vi "ABB configure Bearing run.vi"() -> ()   [LabVIEW 2017]
uses:
  Temp error msg.ctl
  ABB global.vi
panel:
  in  "Temp error":T1="Error: Temperature measurement "
  in  "Category":T2(ring)
  in  "delete reading":bool
  in  "Add reading":bool
  in  "Temperature Measurement channels":i32(listbox)
  in  "Temperature Readings":i32(listbox)
  in  "Auto Reading":T3={"Thermal Stability (°C/hr)"=2.0, "Reading interval (mins)"=2.0}
  in  "Exit":bool
  # "Configure Bearing Run"
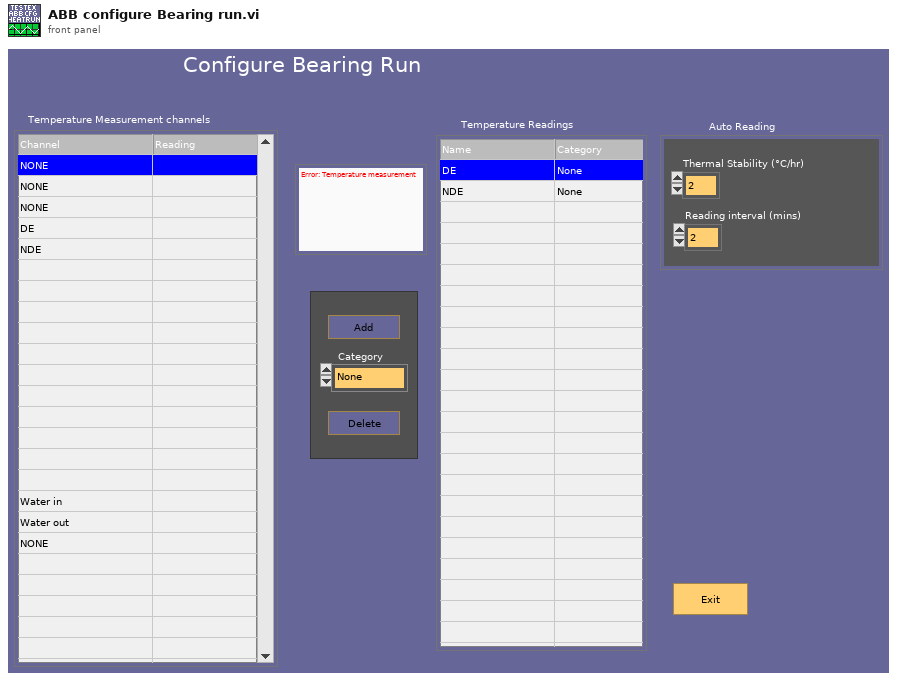
[diagram p1: front panel]
types:
  T1 = typedef "Temp error msg.ctl" = string
  T2 = enum16{"None", "Cool in", "Ambient", "DE", "NDE"}
  T3 = cluster{"Thermal Stability (°C/hr)":dbl, "Reading interval (mins)":dbl}
  T4 = cluster{"temp. alloc":i32[], "category":i32[], "Category names":string[], "Category none names":string[]}
  T5 = cluster{"Thermal Stability (%)":dbl, "Reading interval (mins)":dbl}
  T6 = cluster{"Simulate Norma":bool, "Norma 5000 Address":u8, "WebDaq IP Address":string, "Simulate cDAQ":bool}
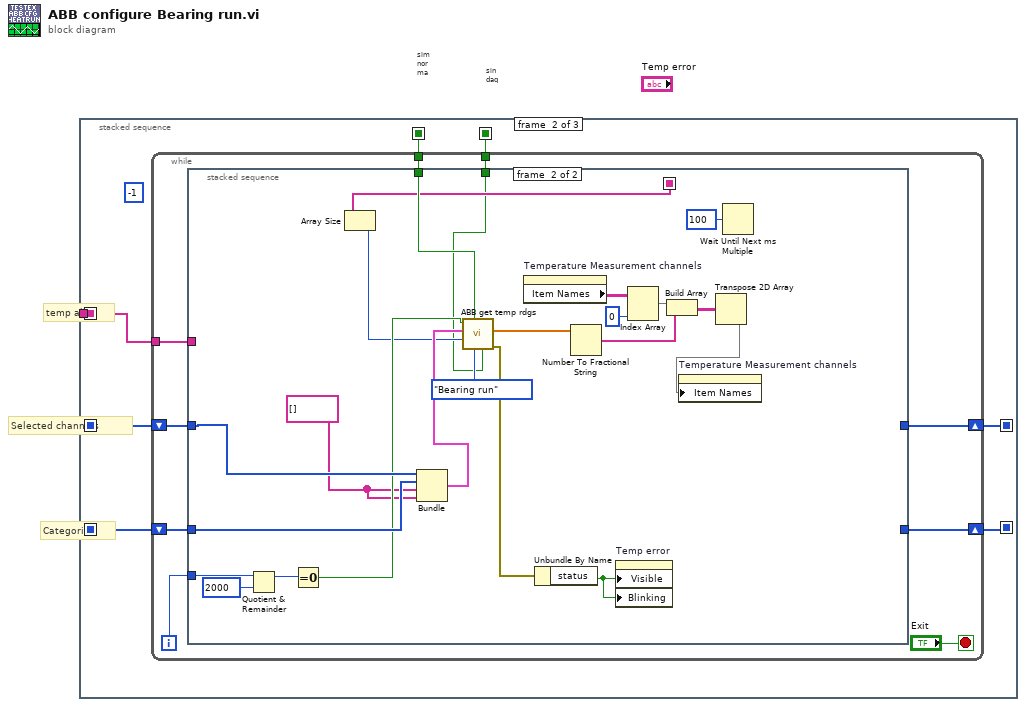
[diagram p0: block diagram]
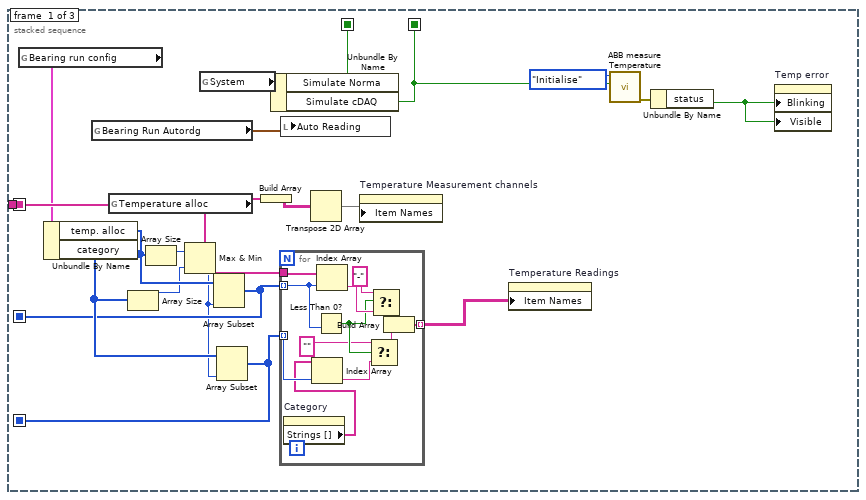
[diagram p2: hidden frame]
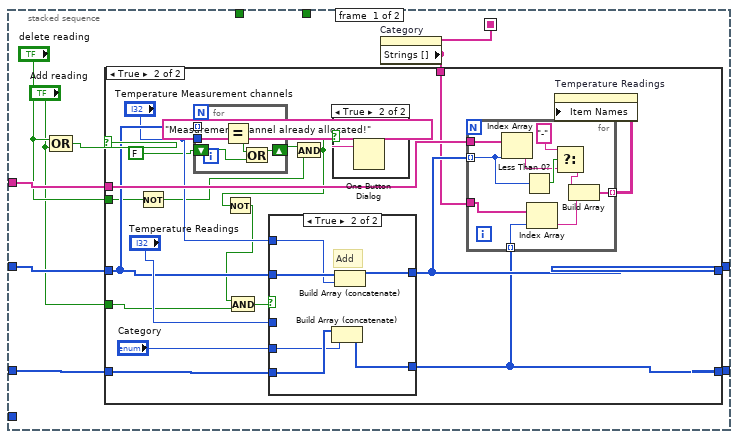
[diagram p3: hidden frame]
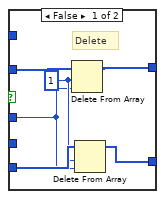
[diagram p6: hidden frame]
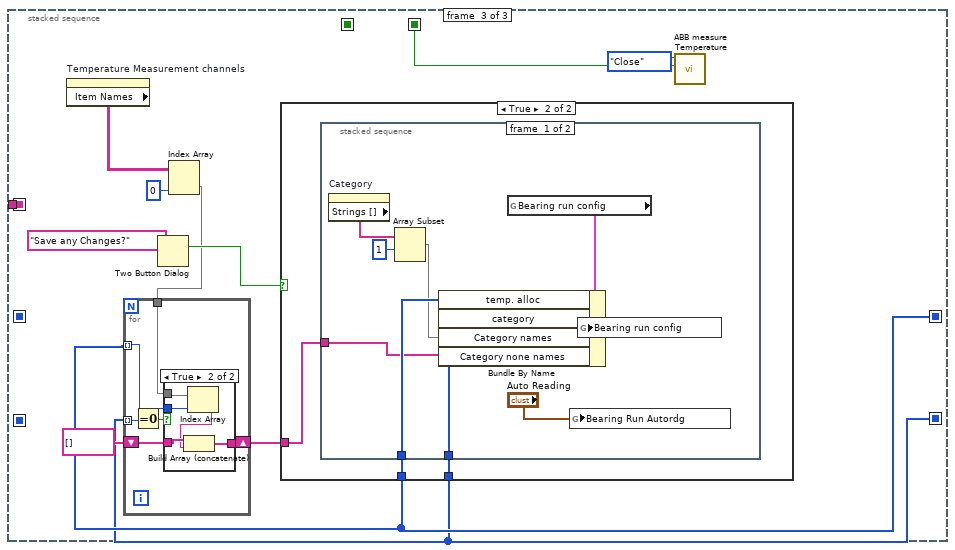
[diagram p7: hidden frame]
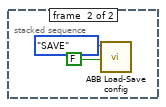
[diagram p10: hidden frame]
diagram:
  # "sin daq"
  # "sim norma"
  # "Categories"
  # "Selected channels"
  # "temp alloc"
  n1 = stacked-sequence {
    seq-local: [w7 _ _] -> [_ w38 _]
    seq-local: [_ w37 _] -> [_ _ w131]
    seq-local: [w16 _ _] -> [_ w36 _]
    seq-local: [w6 _ _] -> [_ w35 _]
    seq-local: [_ w34 _] -> [_ _ w130]
    seq-local: [w12 _ _] -> [_ w33 _]
    seq-local: [w4 _ _] -> [_ w32 w128]
    tunnel: [w16 _ _] -> _
    frame #0 {
      n2 = global read "ABB global.vi" "Bearing run config"() -> (w15:T4)
      n3 = Unbundle By Name(w15) -> ("temp. alloc"=w11:i32[], "category"=w10:i32[])
      n4 = global read "ABB global.vi" "Bearing Run Autordg"() -> (w19:T5)
      n5 = global read "ABB global.vi" "Temperature alloc"() -> (w16:string[])
      n6 = Array Size(array=w10) -> (size(s)=w8:i32)
      n7 = Array Size(array=w11) -> (size(s)=w9:i32)
      n8 = Max & Min(x=w9, y=w8) -> (min(x,y)=w5:i32)  [unwired: 1 out]
      n9 = global read "ABB global.vi" "System"() -> (w13:T6)
      n10 = Array Subset(array=w11, length=w5) -> (w7:i32[])  [unwired: 1 in]
      n11 = Array Subset(array=w10, length=w5) -> (w6:i32[])  [unwired: 1 in]
      n12 = Build Array(w16) -> (w18:string[][])
      n13 = Unbundle By Name(w13) -> ("Simulate Norma"=w12:bool, "Simulate cDAQ"=w4:bool)
      n14 = for {
        tunnel: w16 -> [w31]
        tunnel: w7 -> [w28] mode=indexing
        tunnel: w6 -> [w26] mode=indexing
        tunnel: [w21] -> w14 mode=indexing
        n15 = property on="Category" class="Enum (strict)"() -> ("Strings []"=w25:string[])  [unwired: 2 in, 2 out]
        n16 = Index Array(array=w25, index=w26) -> (element=w24:string)
        n17 = Less Than 0?(x=w28) -> (x < 0?=w27:bool)
        n18 = Index Array(array=w31, index=w28) -> (element=w29:string)
        n19 = Select(t="", s=w27, f=w24) -> (s? t:f=w23:string)
        n20 = Select(t="-", s=w27, f=w29) -> (s? t:f=w22:string)
        n21 = Build Array(w22, w23) -> (w21:string[])
      }
      n22 = local write "Auto Reading"(w19) -> ()
      n23 = Transpose 2D Array(2D array=w18) -> (transposed array=w17:string[][])
      n24 = property on="Temperature Measurement channels" class="MCListbox (strict)"("Item Names"=w17) -> ()  [unwired: 2 in, 2 out]
      n25 = property on="Temperature Readings" class="MCListbox (strict)"("Item Names"=w14) -> ()  [unwired: 2 in, 2 out]
      n26 = call "ABB measure Temperature.vi"("Simulate"=w4, "Mode"=enum16{"Initialise", "Read", "Close"}."Initialise") -> ("error out"=w2:errorcluster)  [unwired: 7 in, 2 out]
      n27 = Unbundle By Name(w2) -> ("status"=w1:bool)
      n28 = property on="Temp error" class="Str (strict)"("Blinking"=w1, "Visible"=w1) -> ()  [unwired: 2 in, 2 out]
    }
    frame #1 {
      (unwired) -1 ("Number Values")
      n29 = while {
        shift-right: [w45] -> w37
        shift-left: w38 -> [w46]
        tunnel: w36 -> [w44]
        shift-right: [w42] -> w34
        shift-left: w35 -> [w43]
        tunnel: w33 -> [w41]
        tunnel: w32 -> [w39]
        i -> [w40]
        stop <- "Exit" stop-if-true
        n30 = stacked-sequence {
          seq-local: [w48 _] -> [_ w110]
          tunnel: w46 -> [w56 w125]
          tunnel: [w55 _] -> w45
          tunnel: w44 -> [w54 _]
          tunnel: w43 -> [w51 w126]
          tunnel: [w50 _] -> w42
          tunnel: w41 -> [_ w127]
          tunnel: w40 -> [_ w115]
          tunnel: w39 -> [_ w107]
          frame #0 {
            n31 = Compound Arithmetic op=OR("delete reading", "Add reading") -> (w53:bool)
            n32 = property on="Category" class="Enum (strict)"() -> ("Strings []"=w48:string[])  [unwired: 2 in, 2 out]
            n33 = case shown="True" w53 {
              tunnel: w56 -> [w58 w69]
              tunnel: [w58 w73] -> w55
              tunnel: w54 -> [_ w76]
              tunnel: "delete reading" -> [_ w62]
              tunnel: w51 -> [w57 w72]
              tunnel: [w57 w71] -> w50
              tunnel: "Add reading" -> [_ w59]
              tunnel: w48 -> [_ w60]
              frame False {
              }
              frame True {
                n34 = Not(x=w62) -> (.not. x?=w61:bool)
                n35 = for {
                  tunnel: w69 -> [w82] mode=indexing
                  tunnel: "Temperature Measurement channels" -> [w81]
                  shift-right: [w78] -> w65
                  shift-left: FALSE -> [w79]
                  n36 = Equal?(x=w82, y=w81) -> (x = y?=w80:bool)
                  n37 = Or(x=w80, y=w79) -> (x .or. y?=w78:bool)
                }
                n38 = And(x=w65, y=w61) -> (x .and. y?=w63:bool)
                n39 = Not(x=w63) -> (.not. x?=w64:bool)
                n40 = And(x=w64, y=w59) -> (x .and. y?=w66:bool)
                n41 = case shown="True" w66 {
                  tunnel: "Category" -> [_ w90]
                  tunnel: "Temperature Measurement channels" -> [_ w92]
                  tunnel: w69 -> [w88 w94]
                  tunnel: [w87 w93] -> w73
                  tunnel: w72 -> [w86 w91]
                  tunnel: [w85 w89] -> w71
                  tunnel: "Temperature Readings" -> [w83 _]
                  frame False {
                    w84 = 1 ("length")
                    # "Delete"
                    n42 = Delete From Array(array=w88, length=w84, index=w83) -> (array with subset deleted=w87:i32[])  [unwired: 1 out]
                    n43 = Delete From Array(array=w86, length=w84, index=w83) -> (array with subset deleted=w85:i32[])  [unwired: 1 out]
                  }
                  frame True {
                    # "Add"
                    n44 = Build Array (concatenate)(w91, w90) -> (w89:i32[])
                    n45 = Build Array (concatenate)(w94, w92) -> (w93:i32[])
                  }
                }
                n46 = case shown="True" w63 {
                  frame False {
                  }
                  frame True {
                    n47 = One Button Dialog(message="Measurement channel already allocated!") -> ()  [unwired: 1 in, 1 out]
                  }
                }
                n48 = for {
                  tunnel: w73 -> [w103] mode=indexing
                  tunnel: w76 -> [w104]
                  tunnel: w60 -> [w98]
                  tunnel: w71 -> [w99] mode=indexing
                  tunnel: [w95] -> w75 mode=indexing
                  n49 = Index Array(array=w104, index=w103) -> (element=w101:string)
                  n50 = Less Than 0?(x=w103) -> (x < 0?=w102:bool)
                  n51 = Index Array(array=w98, index=w99) -> (element=w96:string)
                  n52 = Select(t="-", s=w102, f=w101) -> (s? t:f=w97:string)
                  n53 = Build Array(w97, w96) -> (w95:string[])
                }
                n54 = property on="Temperature Readings" class="MCListbox (strict)"("Item Names"=w75) -> ()  [unwired: 2 in, 2 out]
              }
            }
          }
          frame #1 {
            w111 = string[] []
            n55 = Quotient & Remainder(x=w115, y=2000) -> (x-y*floor(x/y)=w113:i32)  [unwired: 1 out]
            n56 = Equal To 0?(x=w113) -> (x = 0?=w112:bool)
            n57 = Array Size(array=w110) -> (size(s)=w109:i32)
            n58 = Bundle(w125, w126, w111, w111) -> (w124:cluster{i32[], i32[], string[], string[]})  [unwired: 1 in]
            n59 = call "ABB get temp rdgs.vi"("Sim daq"=w107, "sim type"=enum16{"Heat run", "Bearing run"}."Bearing run", "Simulate norma"=w127, "# categories"=w109, "run config"=w124, "start"=w112) -> ("error out"=w106:errorcluster, "Measured temps"=w123:dbl[])  [unwired: 2 in, 2 out]
            n60 = property on="Temperature Measurement channels" class="MCListbox (strict)"() -> ("Item Names"=w122:string[][])  [unwired: 2 in, 2 out]
            n61 = Unbundle By Name(w106) -> ("status"=w105:bool)
            n62 = Number To Fractional String(number=w123) -> (F-format string=w119:string[])  [unwired: 3 in]
            n63 = property on="Temp error" class="Str (strict)"("Visible"=w105, "Blinking"=w105) -> ()  [unwired: 2 in, 2 out]
            n64 = Index Array(array=w122, index (col)=0 ("disabled index (col)")) -> (element=w120:string[])  [unwired: 1 in]
            n65 = Build Array(w120, w119) -> (w118:string[][])
            n66 = Transpose 2D Array(2D array=w118) -> (transposed array=w117:string[][])
            n67 = property on="Temperature Measurement channels" class="MCListbox (strict)"("Item Names"=w117) -> ()  [unwired: 2 in, 2 out]
            n68 = Wait Until Next ms Multiple(millisecond multiple=u32 100) -> ()  [unwired: 1 out]
          }
        }
      }
    }
    frame #2 {
      n69 = property on="Temperature Measurement channels" class="MCListbox (strict)"() -> ("Item Names"=w136:string[][])  [unwired: 2 in, 2 out]
      n70 = Two Button Dialog(message="Save any Changes?") -> (T button?=w138:bool)  [unwired: 2 in]
      n71 = Index Array(array=w136, index (col)=0 ("disabled index (col)")) -> (element=w134:string[])  [unwired: 1 in]
      n72 = for {
        tunnel: w131 -> [w141] mode=indexing
        tunnel: w130 -> [w143] mode=indexing
        tunnel: w134 -> [w142]
        shift-right: [w139] -> w132
        shift-left: string[] [] -> [w140]
        n73 = Equal To 0?(x=w143) -> (x = 0?=w144:bool)
        n74 = case shown="True" w144 {
          tunnel: w142 -> [_ w150]
          tunnel: w141 -> [_ w149]
          tunnel: [w145 w148] -> w139
          tunnel: w140 -> [w145 w147]
          frame False {
          }
          frame True {
            n75 = Index Array(array=w150, index=w149) -> (element=w146:string)
            n76 = Build Array (concatenate)(w147, w146) -> (w148:string[])
          }
        }
      }
      n77 = case shown="True" w138 {
        tunnel: w131 -> [_ w153]
        tunnel: w130 -> [_ w152]
        tunnel: w132 -> [_ w151]
        frame False {
        }
        frame True {
          n78 = stacked-sequence {
            tunnel: w153 -> [w161 _]
            tunnel: w152 -> [w159 _]
            tunnel: w151 -> [w157 _]
            frame #0 {
              n79 = property on="Category" class="Enum (strict)"() -> ("Strings []"=w155:string[])  [unwired: 2 in, 2 out]
              n80 = Array Subset(array=w155, index=1) -> (w156:string[])  [unwired: 1 in]
              n81 = global read "ABB global.vi" "Bearing run config"() -> (w162:T4)
              n82 = Bundle By Name(cluster=w162, "temp. alloc"=w161, "category"=w159, "Category names"=w156, "Category none names"=w157) -> (w160:T4)
              n83 = global write "ABB global.vi" "Bearing Run Autordg"("Auto Reading") -> ()
              n84 = global write "ABB global.vi" "Bearing run config"(w160) -> ()
            }
            frame #1 {
              n85 = call "ABB Load-Save config.vi"("confirm save"=FALSE, "Mode"=enum16{"LOAD", "SAVE"}."SAVE") -> ()  [unwired: 10 in]
            }
          }
        }
      }
      n86 = call "ABB measure Temperature.vi"("Simulate"=w128, "Mode"=enum16{"Initialise", "Read", "Close"}."Close") -> ()  [unwired: 7 in, 3 out]
    }
  }
